vi "X-Y Tracking.vi"(10 "Y Voltage":dbl, 11 "X Voltage":dbl) -> (0 "gave up?":bool, 1 "Y Gauss Amplitude":dbl, 2 "Y centered Voltage":dbl, 3 "X Centered Voltage":dbl, 4 "Cross Section Y":dbl[](graph), 5 "Center Y":dbl, 6 "Cross Section X":dbl[](graph), 7 "Center X":dbl)   [LabVIEW 2012]
uses:
  <vilib>/Analysis/NI_AALPro.lvlib
panel:
  out "amplitude":dbl
  out "Waveform Graph":dbl[](graph)
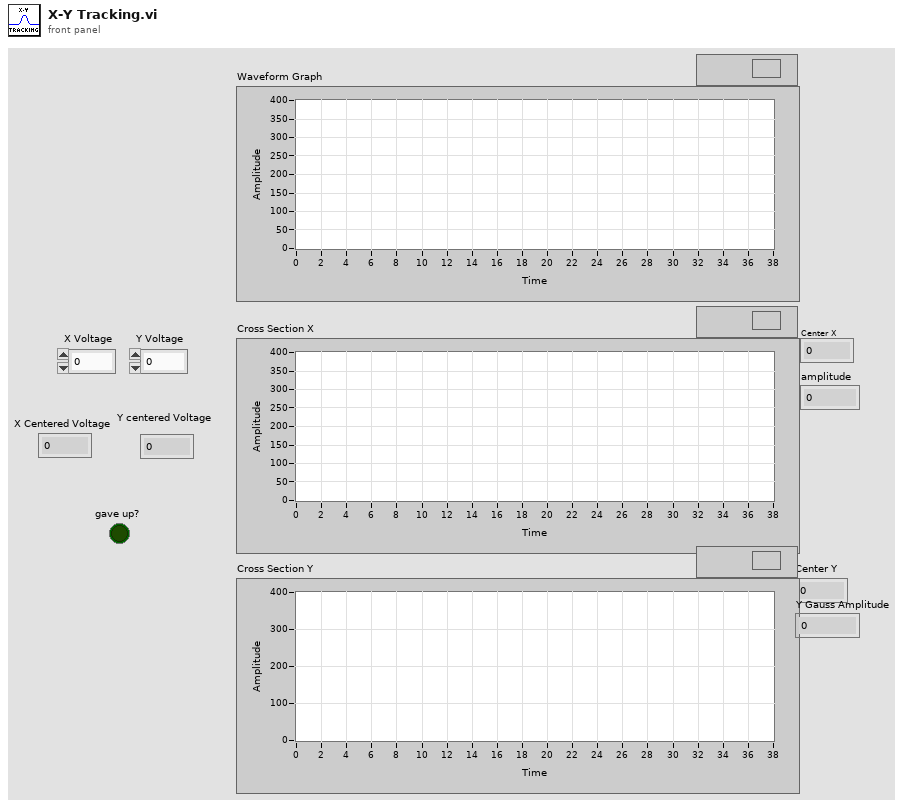
[diagram p1: front panel]
types:
  T1 = cluster{"Number of Y Steps":i32, "Max Y (V)":dbl, "Min Y (V)":dbl}
  T2 = cluster{"Number of X Steps":i32, "Max X (V)":dbl, "Min X (V)":dbl}
  T3 = cluster{"amp min":dbl, "amp max":dbl, "center min":dbl, "center max":dbl, "deviation min":dbl, "deviation max":dbl, "offset min":dbl, "offset max":dbl}
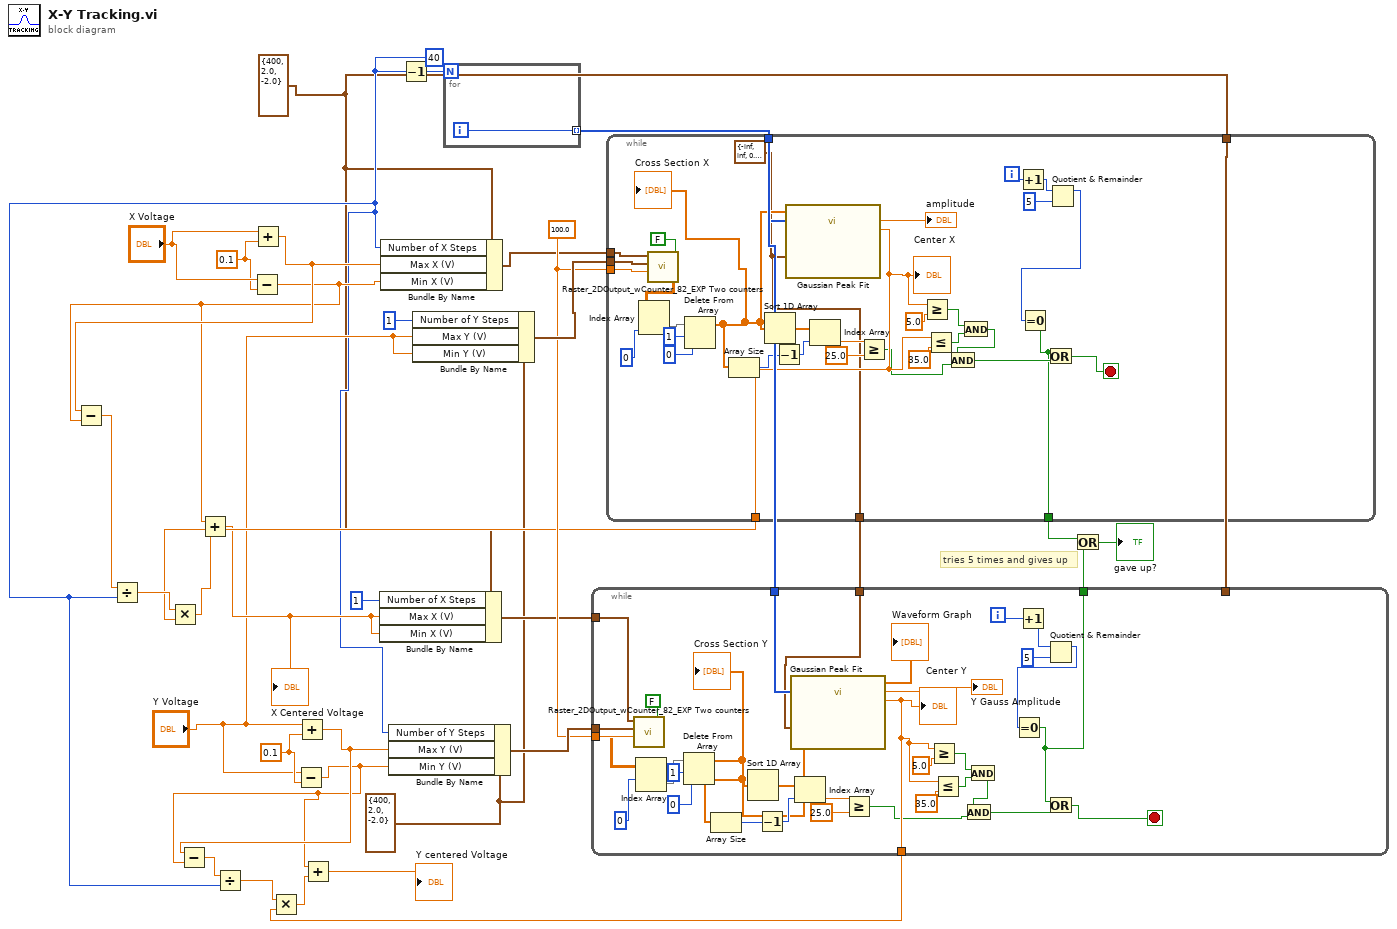
[diagram p0: block diagram]
diagram:
  w16 = 0.1 ("y")
  w17 = T1 {"Number of Y Steps"=400, "Max Y (V)"=2.0, "Min Y (V)"=-2.0} ("Y Parameters")
  w20 = 0.1 ("y")
  w6 = T2 {"Number of X Steps"=400, "Max X (V)"=2.0, "Min X (V)"=-2.0} ("X Parameters")
  w11 = 40 ("Number of X Steps")
  w29 = 100.0 ("Update Rate (Hz)")
  # "tries 5 times and gives up"
  n1 = Subtract(x="X Voltage", y=w20) -> (x-y=w18:dbl)
  n2 = Add(x="X Voltage", y=w20) -> (x+y=w19:dbl)
  n3 = Subtract(x=w19, y=w18) -> (x-y=w28:dbl)
  n4 = Divide(x=w28, y=w11) -> (x/y=w27:dbl)
  n5 = Subtract(x="Y Voltage", y=w16) -> (x-y=w7:dbl)
  n6 = Add(x="Y Voltage", y=w16) -> (x+y=w8:dbl)
  n7 = Subtract(x=w8, y=w7) -> (x-y=w14:dbl)
  n8 = Divide(x=w14, y=w11) -> (x/y=w13:dbl)
  n9 = Bundle By Name(cluster=w6, "Number of X Steps"=w11, "Max X (V)"=w19, "Min X (V)"=w18) -> (w23:T2)
  n10 = Bundle By Name(cluster=w17, "Number of Y Steps"=w11, "Max Y (V)"=w8, "Min Y (V)"=w7) -> (w31:T1)
  n11 = Decrement(x=w11) -> (x-1=w5:i32)
  n12 = Bundle By Name(cluster=w17, "Number of Y Steps"=1, "Max Y (V)"="Y Voltage", "Min Y (V)"="Y Voltage") -> (w32:T1)
  n13 = for {
    N: w5 -> [_]
    tunnel: [w35] -> w34 mode=indexing
    i -> [w35]
  }
  n14 = while {
    tunnel: w34 -> [w65]
    tunnel: w32 -> [w57]
    tunnel: w29 -> [w64]
    tunnel: [w62] -> w26
    tunnel: w23 -> [w58]
    tunnel: w6 -> [_]
    tunnel: [w40] -> w4
    tunnel: [w39] -> w1
    i -> [w48]
    stop <- w41 stop-if-true
    w39 = T3 {"amp min"=-inf, "amp max"=inf, "center min"=0.0, "center max"=45.0, "deviation min"=-inf, "deviation max"=inf, "offset min"=0.0, "offset max"=0.0} ("parameter bounds")
    n15 = call "Raster_2DOutput_wCounter_82_EXP Two counters.vi"("Save?"=FALSE, "Update Rate (Hz)"=w64, "Y Parameters"=w57, "X Parameters"=w58) -> ("Intensity Graph"=w66:dbl[][])  [unwired: 4 in, 1 out]
    n16 = Index Array(array=w66, index (col)=0 ("index (row)")) -> (element=w45:dbl[])  [unwired: 1 in]
    n17 = Delete From Array(array=w45, length=1, index=0) -> (array with subset deleted=w44:dbl[])  [unwired: 1 out]
    "Cross Section X" <- w44
    n18 = Array Size(array=w44) -> (size(s)=w52:i32)
    n19 = Sort 1D Array(array=w44) -> (sorted array=w56:dbl[])
    n20 = Decrement(x=w52) -> (x-1=w51:i32)
    n21 = call <vilib>:"Gaussian Peak Fit.vi"("Y"=w44, "X"=w65, "parameter bounds"=w39) -> ("amplitude"=→"amplitude":dbl, "center"=w62:dbl)  [unwired: 6 in, 5 out]
    "Center X" <- w62
    n22 = Index Array(array=w56, index=w51) -> (element=w55:dbl)
    n23 = Greater Or Equal?(x=w55, y=25.0) -> (x >= y?=w53:bool)
    n24 = Greater Or Equal?(x=w62, y=5.0) -> (x >= y?=w59:bool)
    n25 = Less Or Equal?(x=w62, y=35.0) -> (x <= y?=w60:bool)
    n26 = And(x=w59, y=w60) -> (x .and. y?=w47:bool)
    n27 = And(x=w47, y=w53) -> (x .and. y?=w43:bool)
    n28 = Increment(x=w48) -> (x+1=w49:i32)
    n29 = Quotient & Remainder(x=w49, y=5) -> (x-y*floor(x/y)=w42:i32)  [unwired: 1 out]
    n30 = Equal To 0?(x=w42) -> (x = 0?=w40:bool)
    n31 = Or(x=w40, y=w43) -> (x .or. y?=w41:bool)
  }
  n32 = Multiply(x=w27, y=w26) -> (x*y=w25:dbl)
  n33 = Add(x=w18, y=w25) -> (x+y=w24:dbl)
  "X Centered Voltage" <- w24
  n34 = Bundle By Name(cluster=w6, "Number of X Steps"=1 ("Number of Y Steps"), "Max X (V)"=w24, "Min X (V)"=w24) -> (w22:T2)
  n35 = while {
    tunnel: w34 -> [w100]
    tunnel: w31 -> [w91]
    tunnel: w29 -> [w99]
    tunnel: w22 -> [w92]
    tunnel: [w90] -> w10
    tunnel: w6 -> [_]
    tunnel: [w73] -> w3
    tunnel: w1 -> [w71]
    i -> [w80]
    stop <- w74 stop-if-true
    n36 = call "Raster_2DOutput_wCounter_82_EXP Two counters.vi"("Save?"=FALSE, "Update Rate (Hz)"=w99, "Y Parameters"=w91, "X Parameters"=w92) -> ("Intensity Graph"=w98:dbl[][])  [unwired: 4 in, 1 out]
    n37 = Index Array(array=w98, index (row)=0) -> (element=w77:dbl[])  [unwired: 1 in]
    n38 = Delete From Array(array=w77, length=1, index=0) -> (array with subset deleted=w76:dbl[])  [unwired: 1 out]
    "Cross Section Y" <- w76
    n39 = Array Size(array=w76) -> (size(s)=w84:i32)
    n40 = Sort 1D Array(array=w76) -> (sorted array=w89:dbl[])
    n41 = Decrement(x=w84) -> (x-1=w83:i32)
    n42 = call <vilib>:"Gaussian Peak Fit.vi"("Y"=w76, "X"=w100, "parameter bounds"=w71) -> ("Best Gaussian Fit"=→"Waveform Graph":dbl[], "amplitude"=→"Y Gauss Amplitude":dbl, "center"=w90:dbl)  [unwired: 6 in, 4 out]
    "Center Y" <- w90
    n43 = Index Array(array=w89, index=w83) -> (element=w88:dbl)
    n44 = Greater Or Equal?(x=w88, y=25.0) -> (x >= y?=w85:bool)
    n45 = Greater Or Equal?(x=w90, y=5.0) -> (x >= y?=w96:bool)
    n46 = Less Or Equal?(x=w90, y=35.0) -> (x <= y?=w95:bool)
    n47 = And(x=w96, y=w95) -> (x .and. y?=w86:bool)
    n48 = And(x=w86, y=w85) -> (x .and. y?=w75:bool)
    n49 = Increment(x=w80) -> (x+1=w79:i32)
    n50 = Quotient & Remainder(x=w79, y=5) -> (x-y*floor(x/y)=w81:i32)  [unwired: 1 out]
    n51 = Equal To 0?(x=w81) -> (x = 0?=w73:bool)
    n52 = Or(x=w73, y=w75) -> (x .or. y?=w74:bool)
  }
  n53 = Multiply(x=w13, y=w10) -> (x*y=w12:dbl)
  n54 = Add(x=w7, y=w12) -> (x+y=→"Y centered Voltage":dbl)
  n55 = Or(x=w4, y=w3) -> (x .or. y?=→"gave up?":bool)
